vi "Read configuration.vi"(8 "error in":errorcluster, 11 "GPIC Core editor node in":refnum<class "GPIC Core editor node.lvclass">) -> (0 "error out":errorcluster, 2 "configuration":refnum<class "NISE_CEF_serializable configuration.lvclass">, 3 "GPIC Core editor node out":refnum<class "GPIC Core editor node.lvclass">)   [LabVIEW 2017, in "GPIC Core editor node.lvclass"]
uses:
  GPIC Core editor node.lvclass
  <vilib>/NI/Configuration Framework/serializable configuration/NISE_CEF_serializable configuration.lvclass
  GPIC Core editor node.lvclass/GPIC Core editor node.ctl
  module/configuration/GPIC Core configuration.lvclass
  C:/Program Files (x86)/National Instruments/LabVIEW 2017/vi.lib/NI/Configuration Framework/serializable configuration/NISE_CEF_serializable configuration.lvclass
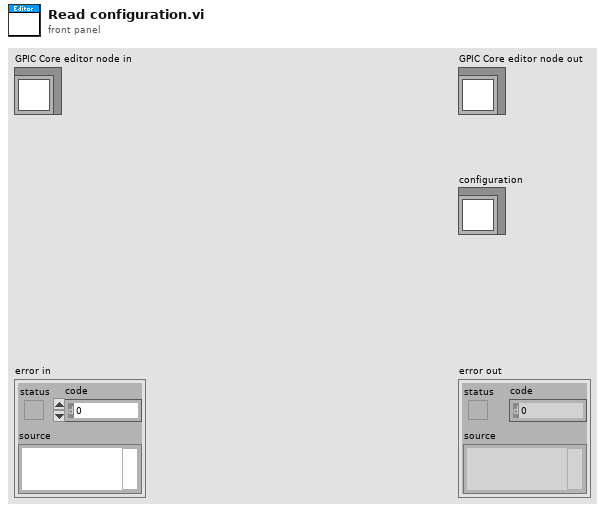
[diagram p1: front panel]
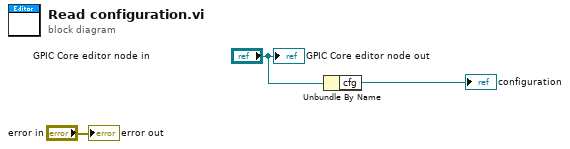
[diagram p0: block diagram]
diagram:
  n1 = Unbundle By Name("GPIC Core editor node in") -> ("cfg"=→"configuration":refnum<class "GPIC Core configuration.lvclass">)
  "error out" <- "error in"
  "GPIC Core editor node out" <- "GPIC Core editor node in"
